vi "CRYFormat Text.vi"(9 "Text Format In":T1, 10 "Text In":string) -> (2 "Text Format Out":T1)   [LabVIEW 2013]
uses:
  Typedef Control/CRYText Format.ctl
panel:
  in  "Font":u16(ring) caption="aa" items=["ADMUI3.fon", "Agency FB", "Agency FB Bold", "Aharoni Bold", "Algerian", "Andalus", "Angsana New", "Angsana New Bold", "Angsana New Bold Italic", "Angsana New Italic", "AngsanaUPC", "AngsanaUPC Bold", "AngsanaUPC Bold Italic", "AngsanaUPC Italic", "Aparajita", "Aparajita Bold", "Aparajita Bold Italic(TrueType)", "Aparajita Italic", "Arabic Typesetting", "Arial", "Arial Black", "Arial Bold", "Arial Bold Italic", "Arial Italic", "Arial Narrow", "Arial Narrow Bold", "Arial Narrow Bold Italic", "Arial Narrow Italic", "Arial Rounded MT Bold", "Arial Unicode MS", "Baskerville Old Face", "Batang & BatangChe & Gungsuh & GungsuhChe", "BatangChe", "Bauhaus 93", "Bell MT", "Bell MT Bold", "Bell MT Italic", "Berlin Sans FB", "Berlin Sans FB Bold", "Berlin Sans FB Demi Bold", "Bernard MT Condensed", "Blackadder ITC", "Bodoni MT", "Bodoni MT Black", "Bodoni MT Black Italic", "Bodoni MT Bold", "Bodoni MT Bold Italic", "Bodoni MT Condensed", "Bodoni MT Condensed Bold", "Bodoni MT Condensed Bold Italic", "Bodoni MT Condensed Italic", "Bodoni MT Italic", "Bodoni MT Poster Compressed", "Book Antiqua", "Book Antiqua Bold", "Book Antiqua Bold Italic", "Book Antiqua Italic", "Bookman Old Style", "Bookman Old Style Bold", "Bookman Old Style Bold Italic", "Bookman Old Style Italic", "Bookshelf Symbol 7", "Bradley Hand ITC", "Britannic Bold", "Broadway", "Browallia New", "Browallia New Bold", "Browallia New Bold Italic", "Browallia New Italic", "BrowalliaUPC", "BrowalliaUPC Bold", "BrowalliaUPC Bold Italic", "BrowalliaUPC Italic", "Brush Script MT Italic", "Calibri", "Calibri Bold", "Calibri Bold Italic", "Calibri Italic", "Californian FB", "Californian FB Bold", "Californian FB Italic", "Calisto MT", "Calisto MT Bold", "Calisto MT Bold Italic", "Calisto MT Italic", "Cambria & Cambria Math", "Cambria Bold", "Cambria Bold Italic", "Cambria Italic", "Candara", "Candara Bold", "Candara Bold Italic", "Candara Italic", "Castellar", "Centaur", "Century", "Century Gothic", "Century Gothic Bold", "Century Gothic Bold Italic", "Century Gothic Italic", "Century Schoolbook", "Century Schoolbook Bold", "Century Schoolbook Bold Italic", "Century Schoolbook Italic", "Chiller", "Colonna MT", "Comic Sans MS", "Comic Sans MS Bold", "Consolas", "Consolas Bold", "Consolas Bold Italic", "Consolas Italic", "Constantia", "Constantia Bold", "Constantia Bold Italic", "Constantia Italic", "Cooper Black", "Copperplate Gothic Bold", "Copperplate Gothic Light", "Corbel", "Corbel Bold", "Corbel Bold Italic", "Corbel Italic", "Cordia New", "Cordia New Bold", "Cordia New Bold Italic", "Cordia New Italic", "CordiaUPC", "CordiaUPC Bold", "CordiaUPC Bold Italic", "CordiaUPC Italic", "Courier 10,12,15", "Courier New", "Courier New Bold", "Courier New Bold Italic", "Courier New Italic", "Curlz MT", "DFKai-SB", "DaunPenh", "David", "David Bold", "DilleniaUPC", "DilleniaUPC Bold", "DilleniaUPC Bold Italic", "DilleniaUPC Italic", "DokChampa", "DotumChe", "Ebrima", "Ebrima Bold", "Edwardian Script ITC", "Elephant", "Elephant Italic", "Engravers MT", "Eras Bold ITC", "Eras Demi ITC", "Eras Light ITC", "Eras Medium ITC", "Estrangelo Edessa", "EucrosiaUPC", "EucrosiaUPC Bold", "EucrosiaUPC Bold Italic", "EucrosiaUPC Italic", "Euphemia", "FangSong", "Felix Titling", "Footlight MT Light", "Forte", "FrankRuehl", "Franklin Gothic Book", "Franklin Gothic Book Italic", "Franklin Gothic Demi", "Franklin Gothic Demi Cond", "Franklin Gothic Demi Italic", "Franklin Gothic Heavy", "Franklin Gothic Heavy Italic", "Franklin Gothic Medium", "Franklin Gothic Medium Cond", "Franklin Gothic Medium Italic", "FreesiaUPC", "FreesiaUPC Bold", "FreesiaUPC Bold Italic", "FreesiaUPC Italic", "Freestyle Script", "French Script MT", "Gabriola", "Garamond", "Garamond Bold", "Garamond Italic", "Gautami", "Gautami Bold", "Georgia", "Georgia Bold", "Georgia Bold Italic", "Georgia Italic", "Gigi", "Gill Sans MT", "Gill Sans MT Bold", "Gill Sans MT Bold Italic", "Gill Sans MT Condensed", "Gill Sans MT Ext Condensed Bold", "Gill Sans MT Italic", "Gill Sans Ultra Bold", "Gill Sans Ultra Bold Condensed", "Gisha", "Gisha Bold", "Gloucester MT Extra Condensed", "Goudy Old Style", "Goudy Old Style Bold", "Goudy Old Style Italic", "Goudy Stout", "Gulim", "Gulim & GulimChe & Dotum & DotumChe", "GulimChe", "Gungsuh", "GungsuhChe", "Haettenschweiler", "Harlow Solid Italic", "Harrington", "High Tower Text", "High Tower Text Italic", "HyhwpEQ", "Impact", "Imprint MT Shadow", "Informal Roman", "IrisUPC", "IrisUPC Bold", "IrisUPC Bold Italic", "IrisUPC Italic", "Iskoola Pota", "Iskoola Pota Bold", "JasmineUPC", "JasmineUPC Bold", "JasmineUPC Bold Italic", "JasmineUPC Italic", "Jokerman", "Juice ITC", "KaiTi", "Kalinga", "Kalinga Bold", "Kartika", "Kartika Bold", "Khmer UI", "Khmer UI Bold", "KodchiangUPC", "KodchiangUPC Bold", "KodchiangUPC Bold Italic", "KodchiangUPC Italic", "Kokila", "Kokila Bold", "Kokila Bold Italic(TrueType)", "Kokila Italic", "Kristen ITC", "Kunstler Script", "Lao UI", "Lao UI Bold", "Latha", "Latha Bold", "Leelawadee", "Leelawadee Bold", "Levenim MT", "Levenim MT Bold", "LilyUPC", "LilyUPC Bold", "LilyUPC Bold Italic", "LilyUPC Italic", "Lucida Bright", "Lucida Bright Demibold", "Lucida Bright Demibold Italic", "Lucida Bright Italic", "Lucida Calligraphy Italic", "Lucida Console", "Lucida Fax Demibold", "Lucida Fax Demibold Italic", "Lucida Fax Italic", "Lucida Fax Regular", "Lucida Handwriting Italic", "Lucida Sans Demibold Italic", "Lucida Sans Demibold Roman", "Lucida Sans Italic", "Lucida Sans Regular", "Lucida Sans Typewriter Bold", "Lucida Sans Typewriter Bold Oblique", "Lucida Sans Typewriter Oblique", "Lucida Sans Typewriter Regular", "Lucida Sans Unicode", "MS Gothic & MS PGothic & MS UI Gothic", "MS Mincho", "MS Mincho & MS PMincho", "MS Outlook", "MS Reference Sans Serif", "MS Reference Specialty", "MS Sans Serif 8,10,12,14,18,24", "MS Serif 8,10,12,14,18,24", "MT Extra", "MV Boli", "Magneto Bold", "Maiandra GD", "Malgun Gothic", "Malgun Gothic Bold", "Mangal", "Mangal Bold", "Matura MT Script Capitals", "Meiryo & Meiryo Italic & Meiryo UI & Meiryo UI Italic", "Meiryo Bold & Meiryo Bold Italic & Meiryo UI Bold & Meiryo UI Bold Italic", "Microsoft Himalaya", "Microsoft JhengHei", "Microsoft JhengHei Bold", "Microsoft New Tai Lue", "Microsoft New Tai Lue Bold", "Microsoft PhagsPa", "Microsoft PhagsPa Bold", "Microsoft Sans Serif", "Microsoft Tai Le", "Microsoft Tai Le Bold", "Microsoft Uighur", "Microsoft YaHei", "Microsoft YaHei Bold", "Microsoft Yi Baiti", "MingLiU & PMingLiU & MingLiU_HKSCS", "MingLiU-ExtB & PMingLiU-ExtB & MingLiU_HKSCS-ExtB", "Miriam", "Miriam Fixed", "Mistral", "Modern", "Modern No. 20", "Mongolian Baiti", "Monotype Corsiva", "MoolBoran", "Narkisim", "NewJumja", "Niagara Engraved", "Niagara Solid", "Nina", "Nina Bold", "Nyala", "OCR A Extended", "Old English Text MT", "Onyx", "Palace Script MT", "Palatino Linotype", "Palatino Linotype Bold", "Palatino Linotype Bold Italic", "Palatino Linotype Italic", "Papyrus", "Parchment", "Perpetua", "Perpetua Bold", "Perpetua Bold Italic", "Perpetua Italic", "Perpetua Titling MT Bold", "Perpetua Titling MT Light", "Plantagenet Cherokee", "Playbill", "Poor Richard", "Pristina", "Raavi", "Raavi Bold", "Rage Italic", "Ravie", "Rockwell", "Rockwell Bold", "Rockwell Bold Italic", "Rockwell Condensed", "Rockwell Condensed Bold", "Rockwell Extra Bold", "Rockwell Italic", "Rod", "Roman", "Sakkal Majalla", "Sakkal Majalla Bold", "Script", "Script MT Bold", "Segoe Print", "Segoe Print Bold", "Segoe Script", "Segoe Script Bold", "Segoe UI", "Segoe UI Bold", "Segoe UI Bold Italic", "Segoe UI Italic", "Segoe UI Light", "Segoe UI Semibold", "Segoe UI Symbol", "Shonar Bangla", "Shonar Bangla Bold", "Showcard Gothic", "Shruti", "Shruti Bold", "SimHei", "SimSun & NSimSun", "SimSun-ExtB", "Simplified Arabic", "Simplified Arabic Bold", "Simplified Arabic Fixed", "Small Fonts", "Small Fonts", "Snap ITC", "Stencil", "Sylfaen", "Symbol", "Tahoma", "Tahoma Bold", "Tempus Sans ITC", "Times New Roman", "Times New Roman Bold", "Times New Roman Bold Italic", "Times New Roman Italic", "Traditional Arabic", "Traditional Arabic Bold", "Trebuchet MS", "Trebuchet MS Bold", "Trebuchet MS Bold Italic", "Trebuchet MS Italic", "Tunga", "Tunga Bold", "Tw Cen MT", "Tw Cen MT Bold", "Tw Cen MT Bold Italic", "Tw Cen MT Condensed", "Tw Cen MT Condensed Bold", "Tw Cen MT Condensed Extra Bold", "Tw Cen MT Italic", "Utsaah", "Utsaah Bold", "Utsaah Bold Italic(TrueType)", "Utsaah Italic", "Vani", "Vani Bold", "Verdana", "Verdana Bold", "Verdana Bold Italic", "Verdana Italic", "Vijaya", "Vijaya Bold", "Viner Hand ITC", "Vivaldi Italic", "Vladimir Script", "Vrinda", "Vrinda Bold", "Webdings", "Wide Latin", "Wingdings", "Wingdings 2", "Wingdings 3"]
  in  "Color":u32(colorbox) caption="aa"
  in  "Cancel":bool
  in  "OK":bool
  out "Text":string
  in  "Strikethrough":bool caption="aa"
  in  "Underline":bool caption="aa"
  in  "Italic":bool caption="aa"
  in  "Bold":bool caption="aa"
  in  "Plain":bool caption="aa"
  in  "Size":u32 caption="aaa"
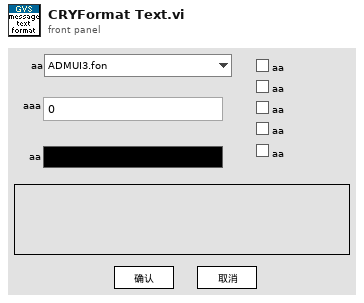
[diagram p1: front panel]
types:
  T1 = typedef "CRYText Format.ctl" = cluster{"Size":u32, "Plain":bool, "Bold":bool, "Italic":bool, "Underline":bool, "Strikethrough":bool, "Color":u32, "Font":string}
  T2 = typedef "GVSText Format.ctl" = cluster{"Size":u32, "Plain":bool, "Bold":bool, "Italic":bool, "Underline":bool, "Strikethrough":bool, "Color":u32, "Font":string}
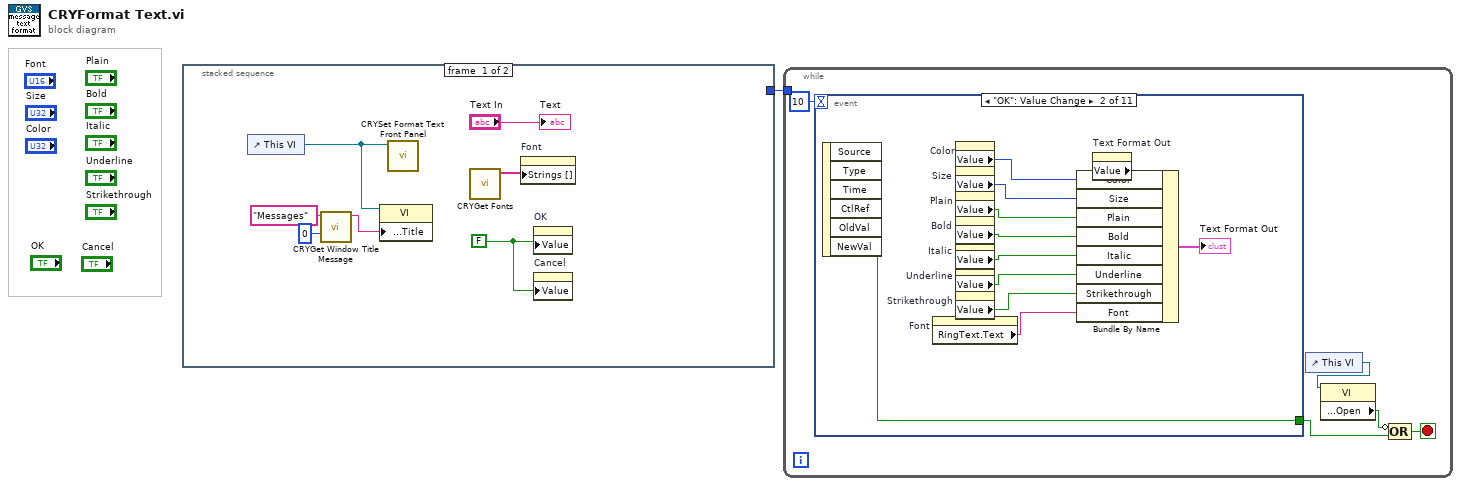
[diagram p0: block diagram]
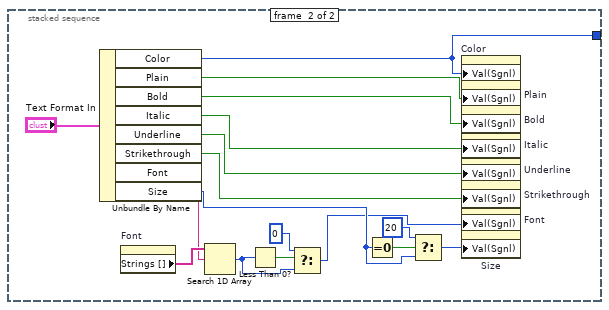
[diagram p2: hidden frame]
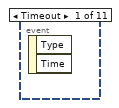
[diagram p3: hidden frame]
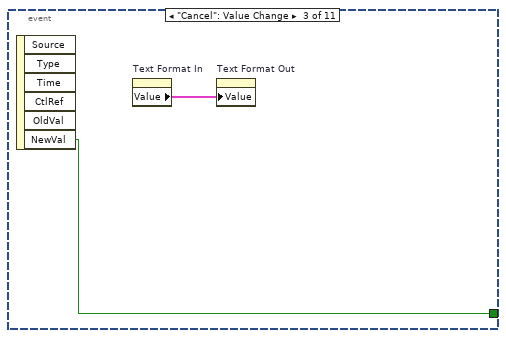
[diagram p4: hidden frame]
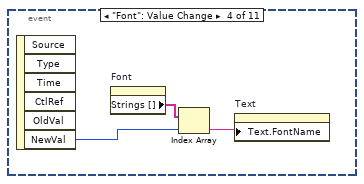
[diagram p5: hidden frame]
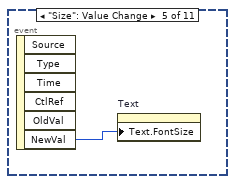
[diagram p6: hidden frame]
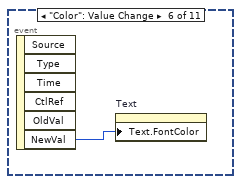
[diagram p7: hidden frame]
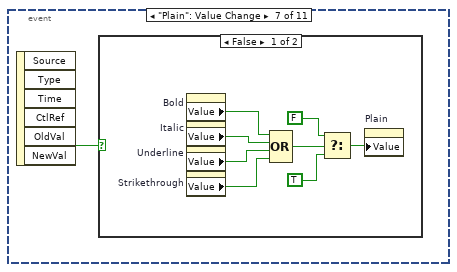
[diagram p8: hidden frame]
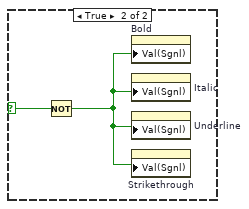
[diagram p9: hidden frame]
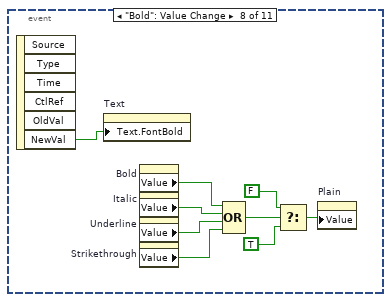
[diagram p10: hidden frame]
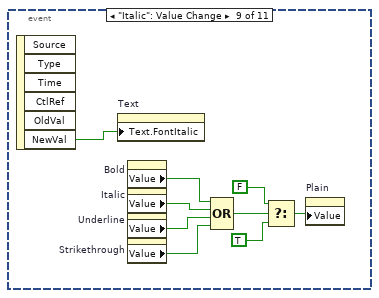
[diagram p11: hidden frame]
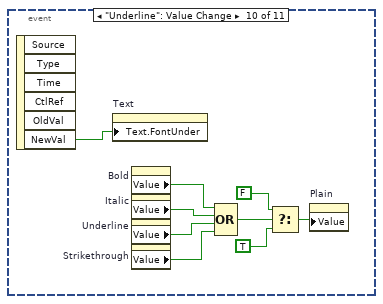
[diagram p12: hidden frame]
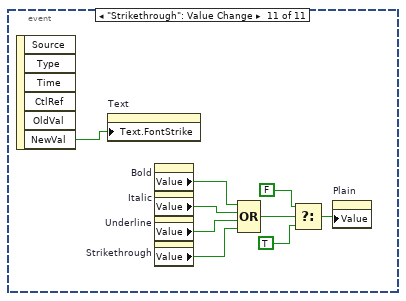
[diagram p13: hidden frame]
diagram:
  n1 = stacked-sequence {
    tunnel: [_ w20] -> w1
    frame #0 {
      w7 = FALSE
      n2 = control-ref of="This VI"() -> (w3:refnum<vi>)
      n3 = call "CRYGet Window Title Message.vi"("No"=0, "Kind"="Messages") -> ("Multibyte String"=w2:string)  [unwired: 4 in, 5 out]
      n4 = property class="VI"(reference=w3, "Front Panel.Title"=w2) -> ()  [unwired: 1 in, 2 out]
      n5 = call "CRYSet Format Text Front Panel.vi"("Vi Ref"=w3) -> ()  [unwired: 11 in]
      n6 = call "CRYGet Fonts.vi"() -> ("Fonts out"=w8:string[])  [unwired: 11 out]
      n7 = property on="Font" class="Ring (strict)"("Strings []"=w8) -> ()  [unwired: 2 in, 2 out]
      n8 = property on="OK" class="Bool (strict)"("Value"=w7) -> ()  [unwired: 2 in, 2 out]
      n9 = property on="Cancel" class="Bool (strict)"("Value"=w7) -> ()  [unwired: 2 in, 2 out]
      "Text" <- "Text In"
    }
    frame #1 {
      n10 = Unbundle By Name("Text Format In") -> ("Color"=w20:u32, "Plain"=w24:bool, "Bold"=w23:bool, "Italic"=w22:bool, "Underline"=w21:bool, "Strikethrough"=w19:bool, "Font"=w13:string, "Size"=w16:u32)
      n11 = property on="Font" class="Ring (strict)"() -> ("Strings []"=w14:string[])  [unwired: 2 in, 2 out]
      n12 = Search 1D Array(1D array=w14, element=w13) -> (index of element=w10:i32)  [unwired: 1 out]
      n13 = Less Than 0?(x=w10) -> (x < 0?=w12:bool)
      n14 = Select(t=u32 0 ("Value (Signaling)"), s=w12, f=w10) -> (s? t:f=w9:u32)
      n15 = Equal To 0?(x=w16) -> (x = 0?=w18:bool)
      n16 = Select(t=u32 20 ("Value (Signaling)"), s=w18, f=w16) -> (s? t:f=w15:u32)
      n17 = property on="Color" class="ColBox"("Val(Sgnl)"=w20) -> ()  [unwired: 2 in, 2 out]
      n18 = property on="Plain" class="Bool (strict)"("Val(Sgnl)"=w24) -> ()  [unwired: 2 in, 2 out]
      n19 = property on="Bold" class="Bool (strict)"("Val(Sgnl)"=w23) -> ()  [unwired: 2 in, 2 out]
      n20 = property on="Italic" class="Bool (strict)"("Val(Sgnl)"=w22) -> ()  [unwired: 2 in, 2 out]
      n21 = property on="Underline" class="Bool (strict)"("Val(Sgnl)"=w21) -> ()  [unwired: 2 in, 2 out]
      n22 = property on="Strikethrough" class="Bool (strict)"("Val(Sgnl)"=w19) -> ()  [unwired: 2 in, 2 out]
      n23 = property on="Font" class="Ring (strict)"("Val(Sgnl)"=w9) -> ()  [unwired: 2 in, 2 out]
      n24 = property on="Size" class="DigNum (strict)"("Val(Sgnl)"=w15) -> ()  [unwired: 2 in, 2 out]
    }
  }
  n25 = while {
    tunnel: w1 -> [_]
    stop <- w26 stop-if-true
    n26 = event shown="[1] \"OK\": Value Change" {
      selector: _ -> [_ _ _ _ _ _ _ _ _ _ _]
      dyn-events: _ -> [_ _ _ _ _ _ _ _ _ _ _]
      timeout: 10 -> [_ _ _ _ _ _ _ _ _ _ _]
      tunnel: [_ w41 w43 _ _ _ _ _ _ _ _] -> w28
      event Timeout {
        n27 = event-data() -> ()  [unwired: 3 out]
      }
      event "OK": Value Change {
        n28 = event-data() -> ("NewVal"=w41:bool)  [unwired: 6 out]
        n29 = property on="Font" class="Ring (strict)"() -> ("RingText.Text"=w31:string)  [unwired: 2 in, 2 out]
        n30 = property on="Color" class="ColBox"() -> ("Value"=w38:u32)  [unwired: 2 in, 2 out]
        n31 = property on="Size" class="DigNum (strict)"() -> ("Value"=w37:u32)  [unwired: 2 in, 2 out]
        n32 = property on="Plain" class="Bool (strict)"() -> ("Value"=w36:bool)  [unwired: 2 in, 2 out]
        n33 = property on="Bold" class="Bool (strict)"() -> ("Value"=w35:bool)  [unwired: 2 in, 2 out]
        n34 = property on="Italic" class="Bool (strict)"() -> ("Value"=w34:bool)  [unwired: 2 in, 2 out]
        n35 = property on="Underline" class="Bool (strict)"() -> ("Value"=w33:bool)  [unwired: 2 in, 2 out]
        n36 = property on="Strikethrough" class="Bool (strict)"() -> ("Value"=w32:bool)  [unwired: 2 in, 2 out]
        n37 = property on="Text Format Out" class="Clust (strict)"() -> ("Value"=w40:T2)  [unwired: 2 in, 2 out]
        n38 = Bundle By Name(cluster=w40, "Color"=w38, "Size"=w37, "Plain"=w36, "Bold"=w35, "Italic"=w34, "Underline"=w33, "Strikethrough"=w32, "Font"=w31) -> (→"Text Format Out":T2)
      }
      event "Cancel": Value Change {
        n39 = event-data() -> ("NewVal"=w43:bool)  [unwired: 6 out]
        n40 = property on="Text Format In" class="Clust (strict)"() -> ("Value"=w42:T2)  [unwired: 2 in, 2 out]
        n41 = property on="Text Format Out" class="Clust (strict)"("Value"=w42) -> ()  [unwired: 2 in, 2 out]
      }
      event "Font": Value Change {
        n42 = event-data() -> ("NewVal"=w46:u16)  [unwired: 6 out]
        n43 = property on="Font" class="Ring (strict)"() -> ("Strings []"=w45:string[])  [unwired: 2 in, 2 out]
        n44 = Index Array(array=w45, index=w46) -> (element=w44:string)
        n45 = property on="Text" class="Str"("Text.FontName"=w44) -> ()  [unwired: 2 in, 2 out]
      }
      event "Size": Value Change {
        n46 = event-data() -> ("NewVal"=w47:u32)  [unwired: 6 out]
        n47 = property on="Text" class="Str"("Text.FontSize"=w47) -> ()  [unwired: 2 in, 2 out]
      }
      event "Color": Value Change {
        n48 = event-data() -> ("NewVal"=w48:u32)  [unwired: 6 out]
        n49 = property on="Text" class="Str"("Text.FontColor"=w48) -> ()  [unwired: 2 in, 2 out]
      }
      event "Plain": Value Change {
        n50 = event-data() -> ("NewVal"=w49:bool)  [unwired: 6 out]
        n51 = case shown="False" w49 {
          selector: w49 -> [_ w59]
          frame False {
            n52 = property on="Bold" class="Bool (strict)"() -> ("Value"=w54:bool)  [unwired: 2 in, 2 out]
            n53 = property on="Italic" class="Bool (strict)"() -> ("Value"=w55:bool)  [unwired: 2 in, 2 out]
            n54 = property on="Underline" class="Bool (strict)"() -> ("Value"=w56:bool)  [unwired: 2 in, 2 out]
            n55 = property on="Strikethrough" class="Bool (strict)"() -> ("Value"=w57:bool)  [unwired: 2 in, 2 out]
            n56 = Compound Arithmetic op=OR(w54, w55, w56, w57) -> (w53:bool)
            n57 = Select(t=FALSE, s=w53, f=TRUE) -> (s? t:f=w50:bool)
            n58 = property on="Plain" class="Bool (strict)"("Value"=w50) -> ()  [unwired: 2 in, 2 out]
          }
          frame True {
            n59 = Not(x=w59) -> (.not. x?=w58:bool)
            n60 = property on="Bold" class="Bool (strict)"("Val(Sgnl)"=w58) -> ()  [unwired: 2 in, 2 out]
            n61 = property on="Italic" class="Bool (strict)"("Val(Sgnl)"=w58) -> ()  [unwired: 2 in, 2 out]
            n62 = property on="Underline" class="Bool (strict)"("Val(Sgnl)"=w58) -> ()  [unwired: 2 in, 2 out]
            n63 = property on="Strikethrough" class="Bool (strict)"("Val(Sgnl)"=w58) -> ()  [unwired: 2 in, 2 out]
          }
        }
      }
      event "Bold": Value Change {
        n64 = event-data() -> ("NewVal"=w68:bool)  [unwired: 6 out]
        n65 = property on="Text" class="Str"("Text.FontBold"=w68) -> ()  [unwired: 2 in, 2 out]
        n66 = property on="Bold" class="Bool (strict)"() -> ("Value"=w60:bool)  [unwired: 2 in, 2 out]
        n67 = property on="Italic" class="Bool (strict)"() -> ("Value"=w61:bool)  [unwired: 2 in, 2 out]
        n68 = property on="Underline" class="Bool (strict)"() -> ("Value"=w62:bool)  [unwired: 2 in, 2 out]
        n69 = property on="Strikethrough" class="Bool (strict)"() -> ("Value"=w63:bool)  [unwired: 2 in, 2 out]
        n70 = Compound Arithmetic op=OR(w60, w61, w62, w63) -> (w64:bool)
        n71 = Select(t=FALSE, s=w64, f=TRUE) -> (s? t:f=w67:bool)
        n72 = property on="Plain" class="Bool (strict)"("Value"=w67) -> ()  [unwired: 2 in, 2 out]
      }
      event "Italic": Value Change {
        n73 = event-data() -> ("NewVal"=w77:bool)  [unwired: 6 out]
        n74 = property on="Text" class="Str"("Text.FontItalic"=w77) -> ()  [unwired: 2 in, 2 out]
        n75 = property on="Bold" class="Bool (strict)"() -> ("Value"=w69:bool)  [unwired: 2 in, 2 out]
        n76 = property on="Italic" class="Bool (strict)"() -> ("Value"=w70:bool)  [unwired: 2 in, 2 out]
        n77 = property on="Underline" class="Bool (strict)"() -> ("Value"=w71:bool)  [unwired: 2 in, 2 out]
        n78 = property on="Strikethrough" class="Bool (strict)"() -> ("Value"=w72:bool)  [unwired: 2 in, 2 out]
        n79 = Compound Arithmetic op=OR(w69, w70, w71, w72) -> (w73:bool)
        n80 = Select(t=FALSE, s=w73, f=TRUE) -> (s? t:f=w76:bool)
        n81 = property on="Plain" class="Bool (strict)"("Value"=w76) -> ()  [unwired: 2 in, 2 out]
      }
      event "Underline": Value Change {
        n82 = event-data() -> ("NewVal"=w86:bool)  [unwired: 6 out]
        n83 = property on="Text" class="Str"("Text.FontUnder"=w86) -> ()  [unwired: 2 in, 2 out]
        n84 = property on="Bold" class="Bool (strict)"() -> ("Value"=w78:bool)  [unwired: 2 in, 2 out]
        n85 = property on="Italic" class="Bool (strict)"() -> ("Value"=w79:bool)  [unwired: 2 in, 2 out]
        n86 = property on="Underline" class="Bool (strict)"() -> ("Value"=w80:bool)  [unwired: 2 in, 2 out]
        n87 = property on="Strikethrough" class="Bool (strict)"() -> ("Value"=w81:bool)  [unwired: 2 in, 2 out]
        n88 = Compound Arithmetic op=OR(w78, w79, w80, w81) -> (w82:bool)
        n89 = Select(t=FALSE, s=w82, f=TRUE) -> (s? t:f=w85:bool)
        n90 = property on="Plain" class="Bool (strict)"("Value"=w85) -> ()  [unwired: 2 in, 2 out]
      }
      event "Strikethrough": Value Change {
        n91 = event-data() -> ("NewVal"=w95:bool)  [unwired: 6 out]
        n92 = property on="Text" class="Str"("Text.FontStrike"=w95) -> ()  [unwired: 2 in, 2 out]
        n93 = property on="Bold" class="Bool (strict)"() -> ("Value"=w87:bool)  [unwired: 2 in, 2 out]
        n94 = property on="Italic" class="Bool (strict)"() -> ("Value"=w88:bool)  [unwired: 2 in, 2 out]
        n95 = property on="Underline" class="Bool (strict)"() -> ("Value"=w89:bool)  [unwired: 2 in, 2 out]
        n96 = property on="Strikethrough" class="Bool (strict)"() -> ("Value"=w90:bool)  [unwired: 2 in, 2 out]
        n97 = Compound Arithmetic op=OR(w87, w88, w89, w90) -> (w91:bool)
        n98 = Select(t=FALSE, s=w91, f=TRUE) -> (s? t:f=w94:bool)
        n99 = property on="Plain" class="Bool (strict)"("Value"=w94) -> ()  [unwired: 2 in, 2 out]
      }
    }
    n100 = control-ref of="This VI"() -> (w29:refnum<vi>)
    n101 = property class="VI"(reference=w29) -> ("Front Panel.Open"=w27:bool)  [unwired: 1 in, 2 out]
    n102 = Compound Arithmetic op=OR(invert w27, w28) -> (w26:bool)
  }
